vi "Calibr FGV.vi"(7 "Function":enum16{"Init", "Read", "Write"}(ring)=enum."Write", 8 "error in (no error)":errorcluster, 11 "Calibr in":refnum<class "Calibr.lvclass">) -> (0 "error out":errorcluster, 3 "Calibr out":refnum<class "Calibr.lvclass">)   [LabVIEW 2018, in "Calibr.lvclass"]
uses:
  Calibr.lvclass
  Calibr.lvclass/Calibr.ctl
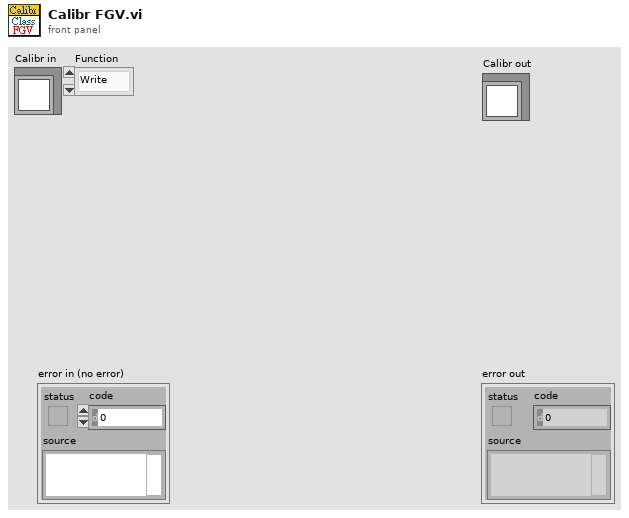
[diagram p1: front panel]
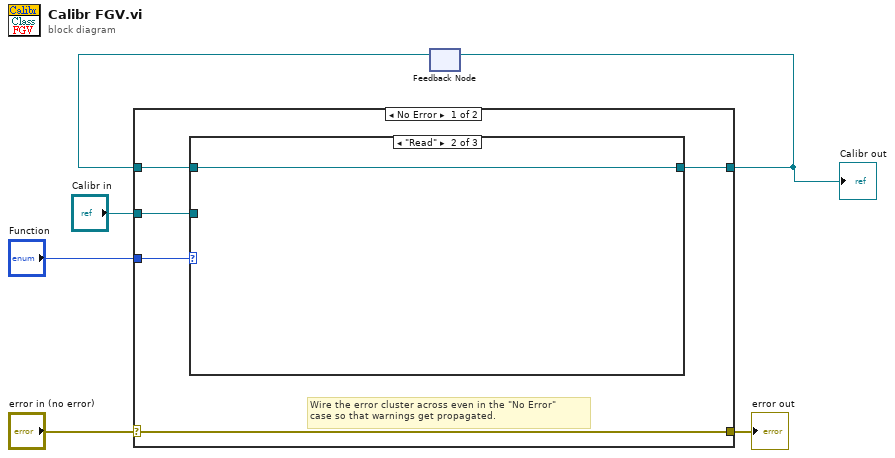
[diagram p0: block diagram]
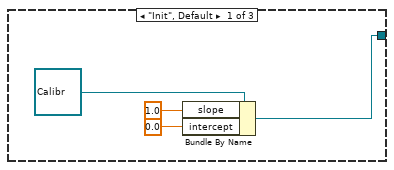
[diagram p2: hidden frame]
diagram:
  n1 = feedback #1() -> (w4:refnum<class "Calibr.lvclass">)  [unwired: 1 in]
  n2 = case shown="No Error" "error in (no error)" {
    selector: "error in (no error)" -> [w11 w19]
    tunnel: [w11 w19] -> w5
    tunnel: [w9 w18] -> w3
    tunnel: w4 -> [w8 w18]
    tunnel: "Function" -> [w10 _]
    tunnel: "Calibr in" -> [w7 _]
    frame No Error {
      # "Wire the error cluster across even in the \"No Error\"\ncase so that warnings get propagated."
      n3 = case shown="\"Read\"" w10 {
        tunnel: [w14 w16 w17] -> w9
        tunnel: w8 -> [_ w16 _]
        tunnel: w7 -> [_ _ w17]
        frame "Init", Default {
          n4 = Bundle By Name(cluster=refnum<class "Calibr.lvclass"> refnum ("Calibr in"), "slope"=1.0, "intercept"=0.0) -> (w14:refnum<class "Calibr.lvclass">)
        }
        frame "Read" {
        }
        frame "Write" {
        }
      }
    }
    frame Error {
    }
  }
  "error out" <- w5
  "Calibr out" <- w3
  n5 = feedback-in #1(w3) -> ()
